vi "Write Boolean Text (UTF-8 String).vi"(8 "error in":errorcluster, 10 "Value":refnum<class "UTF-8 String.lvclass">[](array[class]), 11 "Control Ref":refnum<vi>) -> (0 "error out":errorcluster)   [LabVIEW 2020, in "G-Unicode.lvlib"]
doc: "Write text to a control or indicator, and display it as unicode. <b>Text</b> can be a UTF-8 String or LabVIEW String either as a scalar value, 1D array, or 2D array depending on <b>Control Ref</b> type.\n\nThe <b>Text</b> input also supports UTF-8 Path and LabVIEW Path types, but note that displaying unicode text in a Path control is NOT supported by LabVIEW. Use a string control ref instead.\n\n<b>Note:</b> Tab page text must be manually converted to unicode before programmatic writes will display correctly. To do this, copy and paste existing unicode text into the tab page text for each tab.\n\nSupported control/indicator types and their inputs:\n- String (scalar)\n- String Array (1D)\n- String Array (2D)\n- Ring Text (1D)\n- Tab Pages (1D)\n- Boolean Text (1D, 4 elements)\n- Table (2D)\n- Listbox (1D)\n- Multicolumn Listbox (2D)\n- Graph / Chart Axis Labels (1D, 2 elements)\n- Radio Buttons (1D, 1 element per button)"
uses:
  G-Unicode.lvlib
  Types/UTF-8 String/UTF-8 String.lvclass
  Types/UTF-8 String/UTF-8 String.lvclass/UTF-8 String.ctl
  5206cb6b-04fb-41f5-a37e-29c14f142303.vi
  Private/Conversion/Text as Encoded String.vi
  Private/Conversion/Polymorphic VIs/Text as Encoded String (UTF-8 String).vi
  Types/UTF-8 String/Read Encoded UTF-8 String.vi
  Private/Conversion/Encoded UTF-8 String to Encoded UTF-16LE String.vi
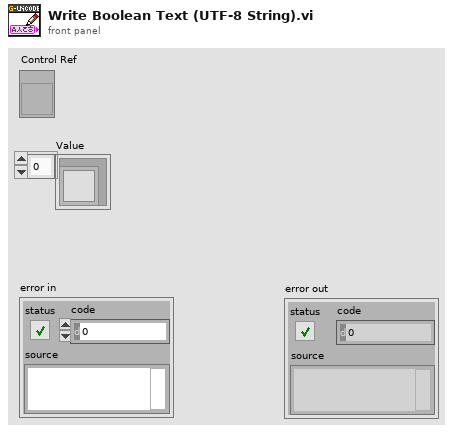
[diagram p1: front panel]
types:
  T1 = typedef "G-Unicode.lvlib/Encoded UTF-16LE String.ctl" = string
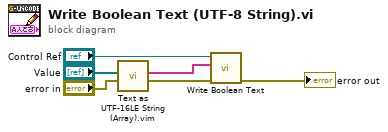
[diagram p0: block diagram]
diagram:
  n1 = call "Text as UTF-16LE String (Array).vim"("error in"="error in", "Text"="Value") -> ("error out"=w1:errorcluster, "Encoded String"=w3:T1[])  [unwired: 8 in]
  n2 = call "Write Boolean Text.vi"("error in"=w1, "Value"=w3, "Boolean Reference in"="Control Ref") -> ("error out"=→"error out":errorcluster)  [unwired: 7 in, 1 out]
